vi "user32_SetActiveWindow.vi"(0 "hWnd":u32, 11 "错误输入（无错误）":errorcluster) -> (4 "dup hWnd":u32, 6 "success?":bool, 8 "hWnd(old)":u32, 15 "错误输出":errorcluster)   [LabVIEW 2011]
doc: "该函数激活一个窗口。该窗口必须与调用线程的消息队列相关联。"
uses:
  user32.dll
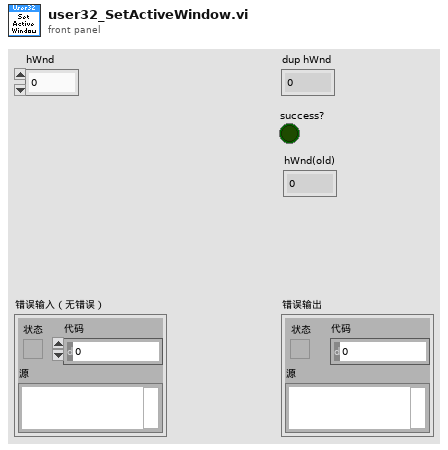
[diagram p1: front panel]
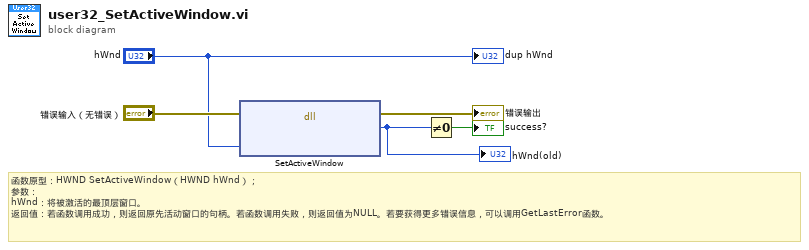
[diagram p0: block diagram]
diagram:
  # "函数原型：HWND SetActiveWindow（HWND hWnd）；\n参数：\nhWnd：将被激活的最顶层窗口。\n返回值：若函数调用成功，则返回原先活动窗口的句柄。若函数调用失败，则返回值为NULL。若要获得更多错误信息，可以调用GetLastError函数。"
  n1 = dll-call lib="user32.dll" fn="SetActiveWindow"(error in="错误输入（无错误）", "hWnd"="hWnd") -> (error out=→"错误输出":errorcluster, "hWnd(old)"=w2:u32)  [unwired: 3 in, 1 out]
  "hWnd(old)" <- w2
  n2 = Not Equal To 0?(x=w2) -> (x != 0?=→"success?":bool)
  "dup hWnd" <- "hWnd"
